vi "Get Display String.vi"(11 "FP GTLT in":refnum<class "FP GTLT.lvclass">) -> (2 "Display String":string)   [LabVIEW 2018, in "FP GTLT.lvclass"]
uses:
  FP GTLT.lvclass
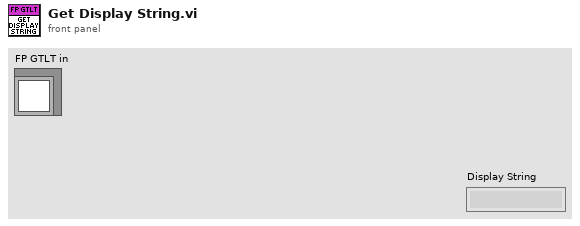
[diagram p1: front panel]
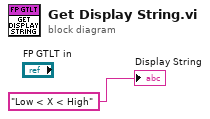
[diagram p0: block diagram]
diagram:
  "Display String" <- "Low < X < High" ("Display String")
